vi "AlliGator Batch Dataset Export Window.vi"() -> ()   [LabVIEW 2021, in "AlliGator Files.lvlib"]
doc: "GUI for batch .ptu datasets export to HDF5 files or folders of TIFF images."
uses:
  AlliGator Files.lvlib
  AlliGator Batch File Conversion Item.ctl
  AlliGator Data Load & Process Options.ctl
  AlliGator Data Information.ctl
  AlliGator Gates to Skip.ctl
  AlliGator Define Gates to.ctl
  AlliGator Gates to Keep.ctl
  AlliGator Gate Arithmetic.ctl
  AlliGator Source Image Settings.ctl
  AlliGator Low Count Pixels Rejection Options.ctl
  AlliGator High Count Pixels Rejection Options.ctl
  AlliGator Image Smoothing Options.ctl
  Arrays/Kernel Type.ctl
  Arrays/Smoothing Algorithm.ctl
  AlliGator Image Binning Options.ctl
  AlliGator Decay Preprocessing Options.ctl
  AlliGator Background Subtraction Parameters.ctl
  AlliGator Baseline Subtraction Method.ctl
  AlliGator Decay Preprocessing Parameters.ctl
  Graphs/XY Graph/XY Graph Plot Shift Parameters.ctl
  Graphs/XY Graph/XY Graph Plot Shift Method.ctl
  <vilib>/Averna/BalloonTip/BalloonTip.llb/BalloonIcon.ctl
  <vilib>/Utility/miscctls.llb/LVPoint32TypeDef.ctl
  <vilib>/Averna/BalloonTip/BalloonTip.llb/OriginPosition.ctl
  AlliGator Variables List.ctl
  AlliGator TIFF Series Options.ctl
  AlliGator Saved TIFF Image Type.ctl
  <vilib>/Averna/BalloonTip/BalloonTip.llb/SetCoords.vi
  835454da-008c-4cc5-9e1e-46d3d2ae4ada.vi
  <vilib>/Averna/BalloonTip/BalloonTip.llb/SetTitle.vi
  <vilib>/Averna/BalloonTip/BalloonTip.llb/SetText.vi
  <vilib>/Averna/BalloonTip/BalloonTip.llb/GetClickEvent.vi
  <vilib>/Averna/BalloonTip/BalloonTip.llb/SetClosable.vi
  <vilib>/Averna/BalloonTip/BalloonTip.llb/SetRoundCorner.vi
  <vilib>/Averna/BalloonTip/BalloonTip.llb/SetBalloonColor.vi
  <vilib>/Averna/BalloonTip/BalloonTip.llb/SetBalloonIcon.vi
  <vilib>/Averna/BalloonTip/BalloonTip.llb/SetCtlRefnum.vi
  <vilib>/Averna/BalloonTip/BalloonTip.llb/SetCtlOriginPosition.vi
  <vilib>/Averna/BalloonTip/BalloonTip.llb/Constructor.vi
  <vilib>/Averna/BalloonTip/BalloonTip.llb/GetDVR.vi
  Variant/Variant to Data/Variant to Boolean.vi
  <userlib>/_OpenG.lib/array/array.llb/Filter 1D Array with Scalar (Boolean)__ogtk.vi
  <userlib>/_OpenG.lib/array/array.llb/Delete Elements from 1D Array (Variant)__ogtk.vi
  <vilib>/ErrorRing/Error Ring.xnode
  GUI/GUI.lvlib
  <userlib>/_OpenG.lib/array/array.llb/openg_array.lvlib
  AlliGator Scripts.lvlib
  AlliGator Decay Analysis.lvlib
  AlliGator Settings.lvlib
  Arrays/Arrays.lvlib
  AlliGator Source Image.lvlib
  AlliGator Decay Preprocessing.lvlib
  Graphs/XY Graph/XY Graph Add-Ons.lvlib
  Notebook/Notebook.lvlib
  Rich Text Box/Rich Text Box.lvlib
  Strings/Strings.lvlib
  AlliGator Globals, Variables & Constants.lvlib
  Variant/Variant to Data/Variant to Data.lvlib
  <vilib>/Averna/BalloonTip/BalloonTip.llb/BalloonTip.lvclass
  Error/Error.lvlib
  Sound/Sound.lvlib
panel:
  out "Conversion Jobs":cluster{"File Path":path, "Exported":bool}[](array[cluster])
  out "Message":string
  out "Animated Busy Icon":bool=TRUE
  in  "Abort":bool
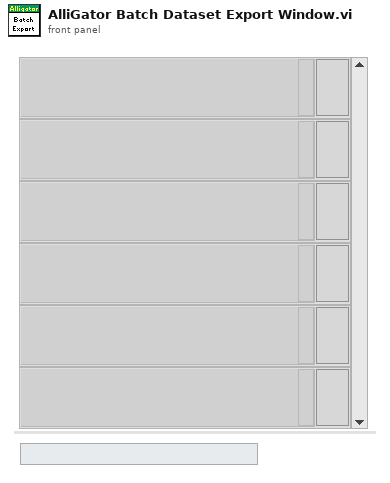
[diagram p1: front panel]
types:
  T1 = enum32{"Invalid", "Standard", "Closed", "Hidden", "Minimized", "Maximized"}
  T2 = typedef "AlliGator Globals, Variables & Constants.lvlib/AlliGator Variables List.ctl" = enum16{"---- GUI ----", "Initialization Status", "State Indicators Refnum", "Original AlliGator Menu Items", "Current Action Loop State", "Script in progress", "Playback", "Loop Playback", "Search ROI Used", "Search ROI", "Decay Graph Max Legend Size", "Intensity Graph Max Legend Size", "Decay Statistics Graph Max Legend Size", "Phasor Graph Max Legend Size", "Phasor Ratio Graph Max Legend Size", "Lifetime Graph Max Legend Size", "---- Files ----", "Export Dataset Frames as Individual Files", "Show Batch Export Help Balloons", "Frames in Dataset", "ptu File Frame Start Indices", "Current Frame in Dataset", "Current Frame Timestamp", "------ Python Plugins ------", "Python Plugins Information", "Python Session", "Valid Python Session?", "---- Source Image ----", "Dataset Loaded", "Dataset Metadata", "Dataset Channel", "Dataset Data Description", "Background Dataset Metadata", "Background Dataset Channel", "Background Dataset Data Description", "Background File Subtraction", "Background File Path", "Background File Pile-up Correction", "Background File Pixel Well Capacity", "Background File Scaling Factor", "Source Image ROIs", "Current Source Image ROI", "Source Image ROI Event Refnum", "X_Source Image Display Range", "X_Source Image Palette Information", "Source Image Palette List", "Source Image Scale", "Current Dataset Load Settings", "Source Image:ROI Overlay Color", "---- Image Profile Window ----", "Image Profile:Overlay ROI in Source Image", "Image Profile Window Event Refnum", "Image Profile:IntensityType", "Image Profile:Intensity Average Type", "Image Profile:Intensity-weighted SDV", "Image Profile:Box Profile Type", "Image Profile Window Open", "Image Profile:Plotted Fit Parameter", "X_Type of Displayed Image", "X_Time Gate Slider", "Dataset Path", "Source Image Overlay to Erase", "Is Displayed Image Accumulated", "White Light Image Modified", "Mask Image Modified", "Macrotime Gate Separation", "------ Phasor Graph -------", "Phasor Graph:Show Line", "---- Phasor Plot ---", "Phasor Plot Parameters Changed", "FLI Dataset Modified since last Phasor Plot Calculation", "Phasor Harmonics Data", "Selected Phasor Harmonics", "Phasor Harmonic Manager Event Refnum", "Phasor Plot ROIs", "Current Phasor Plot ROI", "Phasor Plot ROI Event Refnum", "Phasor Plot Image Reference Points", "Phasor Plot Computed", "Phasor Plot Palette Information", "Phasor Plot Palette List", "Phasor Ratio Palette Information", "Phasor Ratio Palette List", "Phasor Image Scale", "Phasor Plot Image Overlay to Erase", "Phasor Plot Image Elements to Update", "Current Phasor Plot Calculation Parameters", "Current Phasor Calibration Options", "Reset Cumulated Phasor Plot", "Phasor Ratio Reference 1", "Phasor Ratio Lifetime Reference 1", "Phasor Ratio Reference 1 Frequency", "Phasor Ratio Reference 2", "Phasor Ratio Lifetime Reference 2", "Phasor Ratio Reference 2 Frequency", "---- Decay Analysis ----", "Number of Selected Decays to Fit", "LS Fit Results", "LAR Fit Results", "BS Fit Results", "Last Decay Max - Min", "Best Fit Parameters", "Best Fit Parameter Names", "Actual Size X", "Actual Size Y", "Binning X", "Binning Y", "Actual # Gates", "Dataset Number", "Gates to...", "Gates Skipped", "Gates to keep", "Gate Step", "Gate Separation", "Reversed Gates", "Pile-up Correction", "Pixel Well Capacity", "Background Subtracted", "Background Subtraction Method", "Background Definition Range", "Background File (deprecated)", "Number of Dataset Accumulated", "Array of Accumulated Dataset Paths", "Do Averaged Datasets", "Destination File Path", "Process Plot Target", "Use 1/D as Phasor Frequency", "---- Decay Fit Parameter Map -----", "Decay Fit Parameter Map Palette Information", "Decay Fit Parameter Map Palette List", "Local Decay Graph Window Event Refnum", "------- Local Decay Window ---------", "Use normalized IRF for convolution", "----- Miscellaneous ----", "Skippable Dialog Windows Status"}
  T3 = typedef "BalloonTip.lvlib/BalloonTip.lvclass/OriginPosition.ctl" = enum16{"TopLeft", "TopRight", "BottomLeft", "BottomRight"}
  T4 = typedef "LVPoint32TypeDef.ctl" = cluster{"Horizontal":i32, "Vertical":i32}
  T5 = typedef "BalloonTip.lvlib/BalloonTip.lvclass/BalloonIcon.ctl" = enum16{"None", "Information", "Warning", "Error"}
  T6 = typedef "AlliGator Scripts.lvlib/AlliGator Data Load & Process Options.ctl" = cluster{"Data Information":T7, "Source Image Settings":T12, "Decay Preprocessing Options & Parameters":T19, "Clear Phasor Graph":bool}
  T7 = typedef "AlliGator Scripts.lvlib/AlliGator Data Information.ctl" = cluster{"Gates to Skip":T8, "# Gates":u32, "Gate Step":u32, "Gate Duration":dbl[unit], "Gate Separation":dbl[unit], "Pile-up Correction":bool, "Pixel Well Capacity":u32, "Define Gates to":T9, "Gates to Keep":T10, "Laser Period":dbl[unit], "SYNC Period":dbl[unit], "Channel Name":u16, "Channel Arithmetic":T11, "Background File Subtraction":bool, "Background Scaling Factor":dbl, "Background File":path, "Background Pile-up Correction":bool, "Background Pixel Well Capacity":u32, "Dataset Scaling Factor":dbl}
  T8 = typedef "AlliGator Decay Analysis.lvlib/AlliGator Gates to Skip.ctl" = cluster{"Start":u32, "End":u32}
  T9 = typedef "AlliGator Settings.lvlib/AlliGator Define Gates to.ctl" = enum32{"Skip", "Keep"}
  T10 = typedef "AlliGator Settings.lvlib/AlliGator Gates to Keep.ctl" = cluster{"First":u32, "Last":u32}
  T11 = typedef "AlliGator Settings.lvlib/AlliGator Gate Arithmetic.ctl" = enum16{"None", "INT-G2", "G2/INT*<INT>", "(1 - G2/INT)*<INT>"}
  T12 = typedef "AlliGator Scripts.lvlib/AlliGator Source Image Settings.ctl" = cluster{"Low Count Pixels Rejection Options":T13, "High Count Pixels Rejection Options":T14, "Peak Threshold":dbl, "Intensity Threshold":dbl, "Image Smoothing Options":T15, "Image Binning Options":T18}
  T13 = typedef "AlliGator Settings.lvlib/AlliGator Low Count Pixels Rejection Options.ctl" = cluster{"Background Low Threshold Factor":dbl, "Fixed Low Background Threshold":dbl, "Reject Low Count Pixels":bool, "Low Percentile":dbl}
  T14 = typedef "AlliGator Settings.lvlib/AlliGator High Count Pixels Rejection Options.ctl" = cluster{"Background High Threshold Factor":dbl, "Fixed High Background Threshold":dbl, "Reject High Count Pixels":bool, "High Percentile":dbl}
  T15 = typedef "AlliGator Settings.lvlib/AlliGator Image Smoothing Options.ctl" = cluster{"Use Image Smoothing":bool, "Kernel Type":T16, "Bin":i32, "Algorithm":T17}
  T16 = typedef "Arrays.lvlib/Kernel Type.ctl" = enum16{"Uniform", "Bilinear", "Gaussian"}
  T17 = typedef "Arrays.lvlib/Smoothing Algorithm.ctl" = enum16{"Rapid", "Thorough"}
  T18 = typedef "AlliGator Source Image.lvlib/AlliGator Image Binning Options.ctl" = cluster{"Use Image Binning":bool, "X Bin":i32, "Y Bin":i32}
  T19 = typedef "AlliGator Decay Analysis.lvlib/AlliGator Decay Preprocessing.lvlib/AlliGator Decay Preprocessing Options.ctl" = cluster{"Background Subtraction Parameters":T20, "Decay Preprocessing Parameters":T22, "Preprocessing Steps Order":string[]}
  T20 = typedef "AlliGator Decay Analysis.lvlib/AlliGator Decay Preprocessing.lvlib/AlliGator Background Subtraction Parameters.ctl" = cluster{"Background Definition Range":cluster{"Min Gate":dbl[unit], "Max Gate":dbl[unit]}, "Baseline Subtraction Method":T21, "Background Subtraction?":bool, "Background File":path, "Background Constant":dbl, "Background Scaling Factor":dbl, "Background Pile-up Correction":bool, "Background Pixel Well Capacity":u32}
  T21 = typedef "AlliGator Decay Analysis.lvlib/AlliGator Decay Preprocessing.lvlib/AlliGator Baseline Subtraction Method.ctl" = enum16{"Mean", "Min", "Square Gated Single-Exponential", "File", "Constant"}
  T22 = typedef "AlliGator Decay Analysis.lvlib/AlliGator Decay Preprocessing.lvlib/AlliGator Decay Preprocessing Parameters.ctl" = cluster{"Background Subtraction":bool, "Straighten Decay":bool, "Reverse Gates":bool, "1-Normalized Decay":bool, "Smoothen Decay":bool, "Smoothing Parameter":dbl, "Shift Decay":bool, "Decay Shift Parameters":T23, "Extrapolate Decay":bool, "Additional Points":u32, "Head Fraction":dbl, "Pixel-Normalize Decay":bool, "Use Periodicity":bool, "Use Cursors":bool, "Tail Fraction":dbl, "Use Decay Pre-Processing":bool, "Fold Decay":bool, "# Folds":u32, "[0-1]-Normalized Decay":bool}
  T23 = typedef "XY Graph Add-Ons.lvlib/XY Graph Plot Shift Parameters.ctl" = cluster{"Type":T24, "Shift":dbl[unit], "Threshold":dbl, "Rotate":bool}
  T24 = typedef "XY Graph Add-Ons.lvlib/XY Graph Plot Shift Method.ctl" = enum16{"Default", "CFD", "Threshold", "Cross-Correlation"}
  T25 = typedef "AlliGator Files.lvlib/AlliGator Batch File Conversion Item.ctl" = cluster{"File Path":path, "Saved":bool}
  T26 = typedef "LVRectTypeDef.ctl" = cluster{"Left":i16, "Top":i16, "Right":i16, "Bottom":i16}
  T27 = typedef "AlliGator Files.lvlib/AlliGator Saved TIFF Image Type.ctl" = enum16{"Single Gate", "Sum of All Gates", "Phasor"}
  T28 = typedef "AlliGator Files.lvlib/AlliGator TIFF Series Options.ctl" = cluster{"Gate Image File Name":string, "File Number Format":string, "Start Index":u32, "Save Metadata File":bool, "Compress Image":bool}
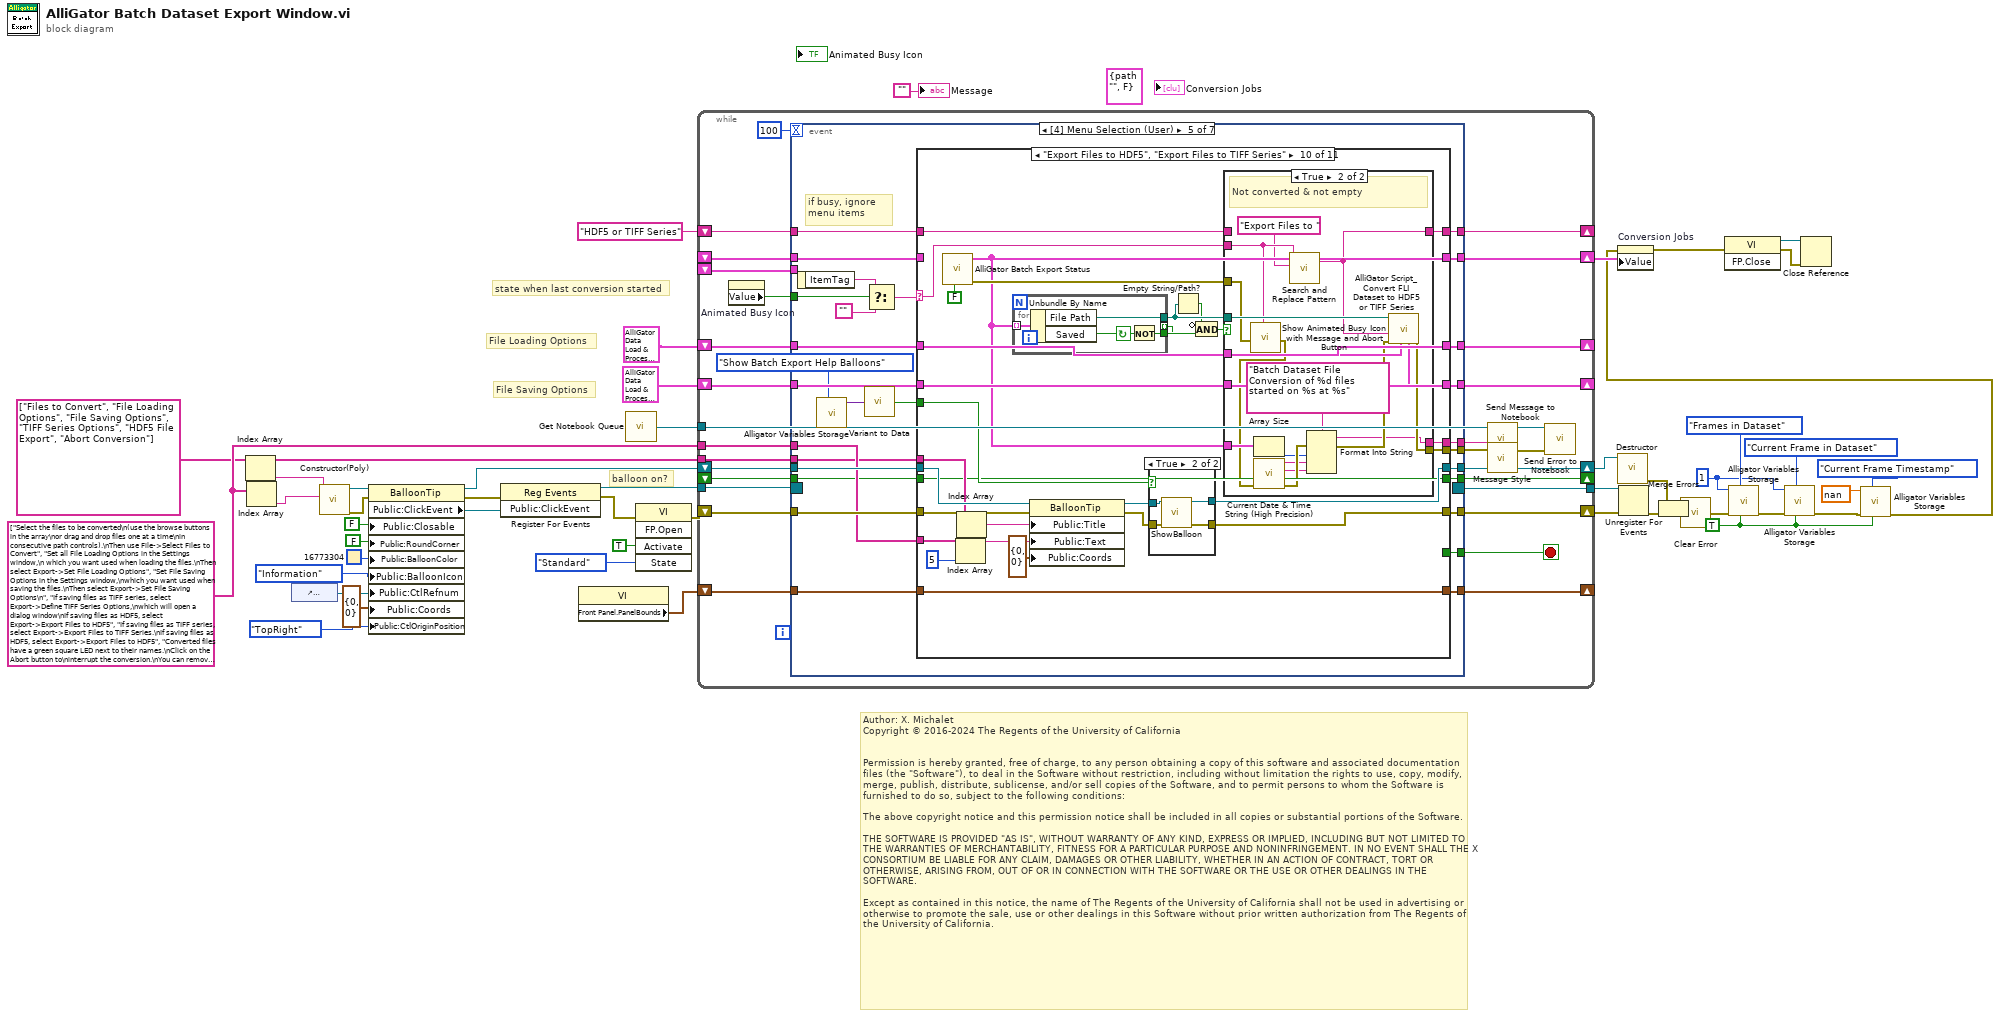
[diagram p0: block diagram]
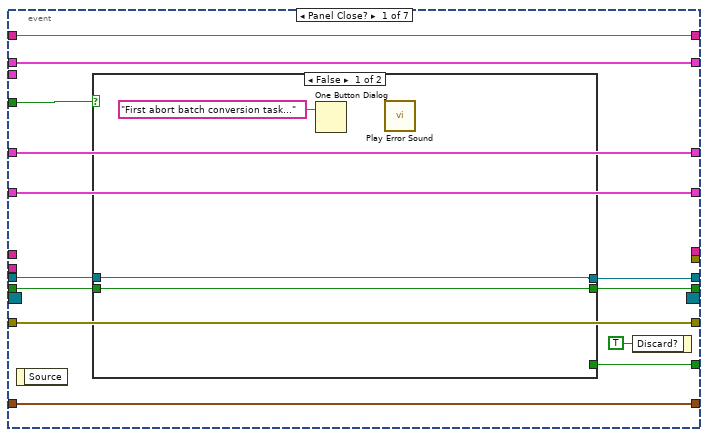
[diagram p2: hidden frame]
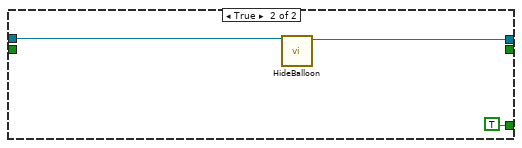
[diagram p3: hidden frame]
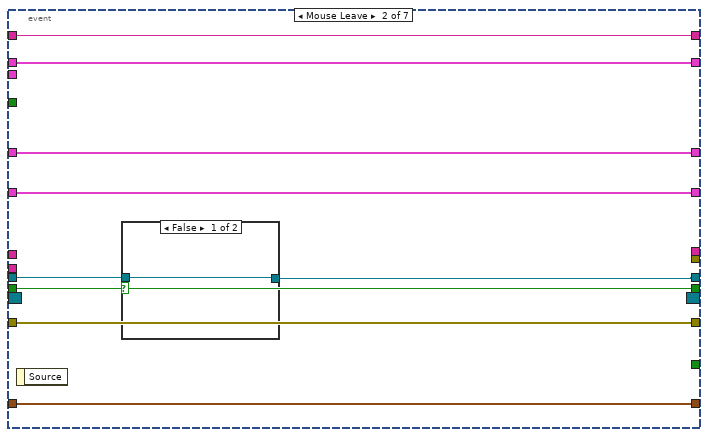
[diagram p4: hidden frame]
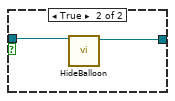
[diagram p5: hidden frame]
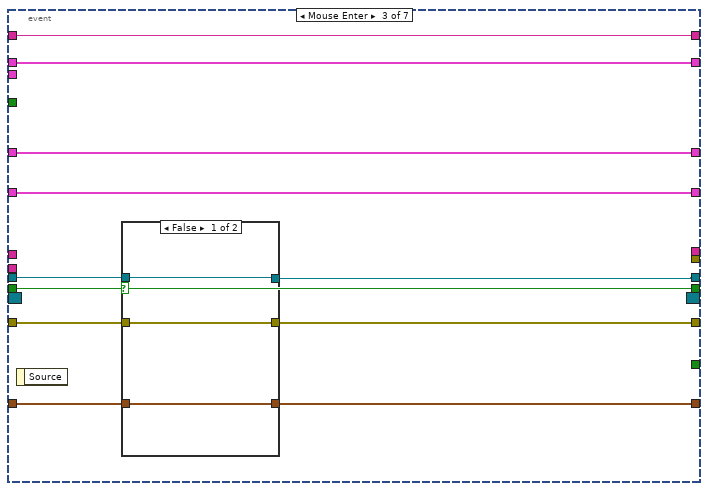
[diagram p6: hidden frame]
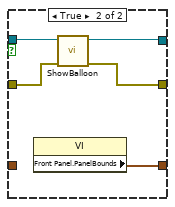
[diagram p7: hidden frame]
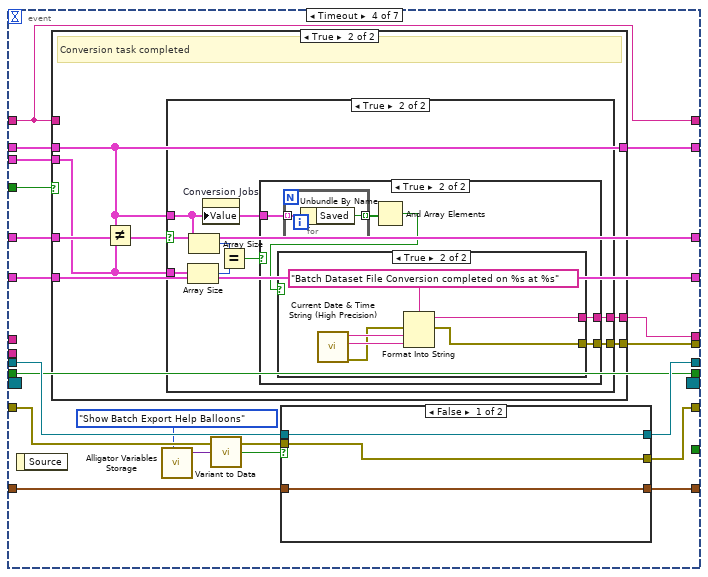
[diagram p8: hidden frame]
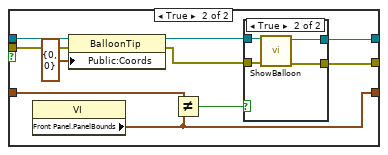
[diagram p9: hidden frame]
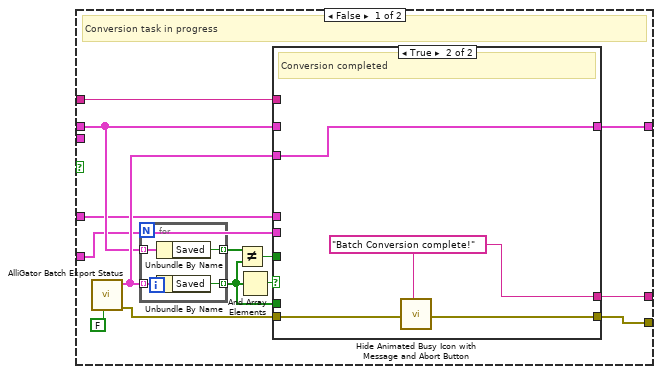
[diagram p11: hidden frame]
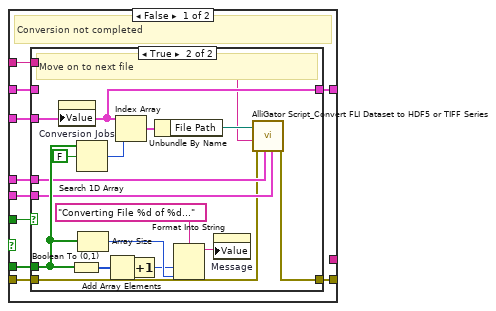
[diagram p12: hidden frame]
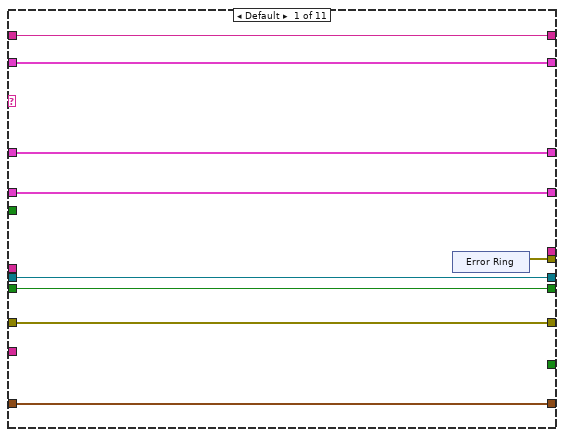
[diagram p17: hidden frame]
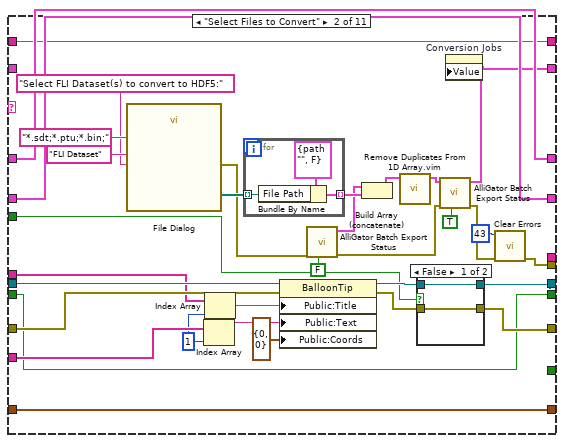
[diagram p18: hidden frame]
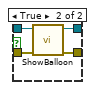
[diagram p19: hidden frame]
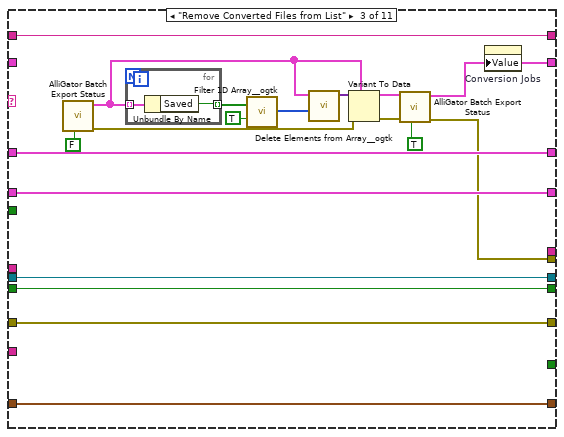
[diagram p20: hidden frame]
diagram:
  w14 = 1
  w11 = TRUE ("Get(F)/Set")
  w29 = string[] ["Files to Convert", "File Loading Options", "File Saving Options", "TIFF Series Options", "HDF5 File Export", "Abort Conversion"]
  w30 = string[] ["Select the files to be converted\n(use the browse buttons in the array\nor drag and drop files one at a time\nin consecutive path controls).\nThen use File->Select Files to Convert", "Set all File Loading Options in the Settings window,\n which you want used when loading the files.\nThen select Export->Set File Loading Options", "Set File Saving Options in the Settings window,\nwhich you want used when saving the files.\nThen select Export->Set File Saving Options\n", "If saving files as TIFF series, select Export->Define TIFF Series Options,\nwhich will open a dialog window\nIf saving files as HDF5, select Export->Export Files to HDF5", "If saving files as TIFF series, select Export->Export Files to TIFF Series.\nIf saving files as HDF5, select Export->Export Files to HDF5", "Converted files have a green square LED next to their names.\nClick on the Abort button to\ninterrupt the conversion.\nYou can remove the converted files\nfrom the list using File->Remove Converted Files from List."] ("Text")
  (unwired) T25 {"File Path"=path "", "Saved"=FALSE} ("File Array")
  # "Author: X. Michalet\nCopyright © 2016-2024 The Regents of the University of California\n \n\nPermission is hereby granted, free of charge, to any person obtaining a copy of this software and associated documentation files (the \"Software\"), to deal in the Software without restriction, including without limitation the rights to use, copy, modify, merge, publish, distribute, sublicense, and/or sell copies of the Software, and to permit persons to whom the Software is furnished to do so, subject to the following conditions:\n\nThe above copyright notice and this permission notice shall be included in all copies or substantial portions of the Software.\n\nTHE SOFTWARE IS PROVIDED \"AS IS\", WITHOUT WARRANTY OF ANY KIND, EXPRESS OR IMPLIED, INCLUDING BUT NOT LIMITED TO THE WARRANTIES OF MERCHANTABILITY, FITNESS FOR A PARTICULAR PURPOSE AND NONINFRINGEMENT. IN NO EVENT SHALL THE X CONSORTIUM BE LIABLE FOR ANY CLAIM, DAMAGES OR OTHER LIABILITY, WHETHER IN AN ACTION OF CONTRACT, TORT OR OTHERWISE, ARISING FROM, OUT OF OR IN CONNECTION WITH THE SOFTWARE OR THE USE OR OTHER DEALINGS IN THE SOFTWARE.\n\nExcept as contained in this notice, the name of The Regents of the University of California shall not be used in advertising or otherwise to promote the sale, use or other dealings in this Software without prior written authorization from The Regents of the University of California."
  # "balloon on?"
  # "File Saving Options"
  # "File Loading Options"
  # "state when last conversion started"
  n1 = Index Array(array=w29) -> (element=w25:string)  [unwired: 1 in]
  n2 = Index Array(array=w30) -> (element=w24:string)  [unwired: 1 in]
  n3 = control-ref of="Conversion Jobs"() -> (w28:refnum<vi>)
  n4 = call-poly <vilib>:"Constructor(Poly).vi"("Text"=w24, "Title (\"\")"=w25) -> ("error out"=w39:errorcluster, "BalloonTip out"=w40:refnum<class "BalloonTip.lvclass">)  [unwired: 8 in]
  n5 = property class="BalloonTip"(reference=w40, error in=w39, "Public:Closable"=FALSE ("Closable"), "Public:RoundCorner"=FALSE ("RoundCorner"), "Public:BalloonColor"=u32 16773304 ("BalloonColor"), "Public:BalloonIcon"=BalloonIcon."Information" ("BalloonIcon"), "Public:CtlRefnum"=w28, "Public:Coords"=T4 {"Horizontal"=0, "Vertical"=0} ("Coords"), "Public:CtlOriginPosition"=OriginPosition."TopRight" ("CtlOriginPosition")) -> (reference out=w38:refnum<class "BalloonTip.lvclass">, error out=w41:errorcluster, "Public:ClickEvent"=w2:refnum<user-event>)
  n6 = register-events(error in=w41, w2) -> (reference out=w37:refnum<event-registration>, error out=w5:errorcluster)  [unwired: 1 in]
  n7 = property class="VI"() -> ("Front Panel.PanelBounds"=w23:T26)  [unwired: 2 in, 2 out]
  n8 = call "Get Notebook Queue.vi"() -> ("Notebook Queue"=w1:refnum<queue>)  [unwired: 9 in]
  n9 = invoke class="VI" method="FP.Open"(error in=w5, "Activate"=TRUE ("Activate?"), "State"=T1."Standard") -> (error out=w6:errorcluster)  [unwired: 2 in, 4 out]
  n10 = while {
    shift-right: [w75] -> w46
    shift-left: _ -> [w73]
    shift-left: _ -> [w74]
    shift-right: [w72] -> _
    shift-left: T6 {"Data Information"={"Gates to Skip"={"Start"=0, "End"=0}, "# Gates"=1, "Gate Step"=1, "Gate Duration"=3e-10, "Gate Separation"=4e-11, "Pile-up Correction"=FALSE, "Pixel Well Capacity"=1, "Define Gates to"=enum."Skip", "Gates to Keep"={"First"=0, "Last"=0}, "Laser Period"=0.0, "SYNC Period"=0.0, "Channel Name"=0, "Channel Arithmetic"=enum."None", "Background File Subtraction"=FALSE, "Background Scaling Factor"=1.0, "Background File"=path "", "Background Pile-up Correction"=FALSE, "Background Pixel Well Capacity"=1, "Dataset Scaling Factor"=1.0}, "Source Image Settings"={"Low Count Pixels Rejection Options"={"Background Low Threshold Factor"=0.0, "Fixed Low Background Threshold"=20000.0, "Reject Low Count Pixels"=FALSE, "Low Percentile"=0.0}, "High Count Pixels Rejection Options"={"Background High Threshold Factor"=0.0, "Fixed High Background Threshold"=1.0, "Reject High Count Pixels"=FALSE, "High Percentile"=100.0}, "Peak Threshold"=500.0, "Intensity Threshold"=500.0, "Image Smoothing Options"={"Use Image Smoothing"=FALSE, "Kernel Type"=enum."Bilinear", "Bin"=1, "Algorithm"=enum."Rapid"}, "Image Binning Options"={"Use Image Binning"=FALSE, "X Bin"=1, "Y Bin"=1}}, "Decay Preprocessing Options & Parameters"={"Background Subtraction Parameters"={"Background Definition Range"={"Min Gate"=0.0, "Max Gate"=0.0}, "Baseline Subtraction Method"=enum."Mean", "Background Subtraction?"=FALSE, "Background File"=path "", "Background Constant"=0.0, "Background Scaling Factor"=1.0, "Background Pile-up Correction"=FALSE, "Background Pixel Well Capacity"=1}, "Decay Preprocessing Parameters"={"Background Subtraction"=FALSE, "Straighten Decay"=FALSE, "Reverse Gates"=FALSE, "1-Normalized Decay"=FALSE, "Smoothen Decay"=FALSE, "Smoothing Parameter"=0.0, "Shift Decay"=FALSE, "Decay Shift Parameters"={"Type"=enum."Default", "Shift"=0.0, "Threshold"=0.0, "Rotate"=FALSE}, "Extrapolate Decay"=FALSE, "Additional Points"=0, "Head Fraction"=0.0, "Pixel-Normalize Decay"=FALSE, "Use Periodicity"=FALSE, "Use Cursors"=FALSE, "Tail Fraction"=0.0, "Use Decay Pre-Processing"=TRUE, "Fold Decay"=FALSE, "# Folds"=1, "[0-1]-Normalized Decay"=FALSE}, "Preprocessing Steps Order"=[]}, "Clear Phasor Graph"=FALSE} ("Dataset Loading & Pre-processing Options (out)") -> [w71]
    shift-right: [w70] -> _
    shift-left: T6 {"Data Information"={"Gates to Skip"={"Start"=0, "End"=0}, "# Gates"=1, "Gate Step"=1, "Gate Duration"=3e-10, "Gate Separation"=4e-11, "Pile-up Correction"=FALSE, "Pixel Well Capacity"=1, "Define Gates to"=enum."Skip", "Gates to Keep"={"First"=0, "Last"=0}, "Laser Period"=0.0, "SYNC Period"=0.0, "Channel Name"=0, "Channel Arithmetic"=enum."None", "Background File Subtraction"=FALSE, "Background Scaling Factor"=1.0, "Background File"=path "", "Background Pile-up Correction"=FALSE, "Background Pixel Well Capacity"=1, "Dataset Scaling Factor"=1.0}, "Source Image Settings"={"Low Count Pixels Rejection Options"={"Background Low Threshold Factor"=0.0, "Fixed Low Background Threshold"=20000.0, "Reject Low Count Pixels"=FALSE, "Low Percentile"=0.0}, "High Count Pixels Rejection Options"={"Background High Threshold Factor"=0.0, "Fixed High Background Threshold"=1.0, "Reject High Count Pixels"=FALSE, "High Percentile"=100.0}, "Peak Threshold"=500.0, "Intensity Threshold"=500.0, "Image Smoothing Options"={"Use Image Smoothing"=FALSE, "Kernel Type"=enum."Bilinear", "Bin"=1, "Algorithm"=enum."Rapid"}, "Image Binning Options"={"Use Image Binning"=FALSE, "X Bin"=1, "Y Bin"=1}}, "Decay Preprocessing Options & Parameters"={"Background Subtraction Parameters"={"Background Definition Range"={"Min Gate"=0.0, "Max Gate"=0.0}, "Baseline Subtraction Method"=enum."Mean", "Background Subtraction?"=FALSE, "Background File"=path "", "Background Constant"=0.0, "Background Scaling Factor"=1.0, "Background Pile-up Correction"=FALSE, "Background Pixel Well Capacity"=1}, "Decay Preprocessing Parameters"={"Background Subtraction"=FALSE, "Straighten Decay"=FALSE, "Reverse Gates"=FALSE, "1-Normalized Decay"=FALSE, "Smoothen Decay"=FALSE, "Smoothing Parameter"=0.0, "Shift Decay"=FALSE, "Decay Shift Parameters"={"Type"=enum."Default", "Shift"=0.0, "Threshold"=0.0, "Rotate"=FALSE}, "Extrapolate Decay"=FALSE, "Additional Points"=0, "Head Fraction"=0.0, "Pixel-Normalize Decay"=FALSE, "Use Periodicity"=FALSE, "Use Cursors"=FALSE, "Tail Fraction"=0.0, "Use Decay Pre-Processing"=TRUE, "Fold Decay"=FALSE, "# Folds"=1, "[0-1]-Normalized Decay"=FALSE}, "Preprocessing Steps Order"=[]}, "Clear Phasor Graph"=FALSE} ("Dataset Loading & Pre-processing Options (out)") -> [w69]
    tunnel: w1 -> [w52]
    shift-right: [w68] -> _
    shift-left: "HDF5 or TIFF Series" ("result string") -> [w67]
    tunnel: w37 -> [w62]
    shift-right: [w61] -> w33
    shift-left: w38 -> [w63]
    tunnel: [w60] -> w32
    shift-right: [w59] -> w31
    shift-left: w6 -> [w64]
    tunnel: w30 -> [w58]
    tunnel: w29 -> [w57]
    shift-right: [w55] -> _
    shift-left: w23 -> [w56]
    shift-right: [w54] -> _
    shift-left: _ -> [w53]
    stop <- w65 stop-if-true
    n11 = property on="Animated Busy Icon" class="Bool (strict)"() -> ("Value"=w66:bool)  [unwired: 2 in, 2 out]
    n12 = event shown="[4] Menu Selection (User)" {
      selector: w62 -> [_ _ _ _ _ _ _]
      dyn-events: [_ _ _ _ _ _ _] -> w60
      timeout: 100 -> [_ _ _ _ _ _ _]
      tunnel: w66 -> [w89 _ _ w145 w268 _ _]
      tunnel: [w87 _ _ _ w266 _ _] -> w65
      tunnel: [w86 w104 w118 w143 w265 w567 w596] -> w75
      tunnel: w74 -> [w86 w104 w118 w144 w264 w567 w596]
      tunnel: w73 -> [_ _ _ w142 _ _ _]
      tunnel: [w85 w103 w117 w141 w261 w576 w595] -> w72
      tunnel: w71 -> [w85 w103 w117 w141 w260 w576 w595]
      tunnel: [w84 w102 w116 w140 w259 w575 w594] -> w70
      tunnel: w69 -> [w84 w102 w116 w140 w258 w575 w594]
      tunnel: [_ _ _ w139 w257 _ w592] -> w49
      tunnel: [w83 w101 w115 w138 w256 w574 w593] -> w68
      tunnel: w67 -> [w83 w101 w115 w138 w255 w574 w593]
      tunnel: w64 -> [w82 w100 w112 w134 w252 w559 w582]
      tunnel: w63 -> [w80 w98 w114 w135 w254 w560 w585]
      tunnel: [w79 w97 w113 w137 w253 w560 w584] -> w61
      tunnel: [w82 w100 w111 w136 w251 w559 w583] -> w59
      tunnel: w58 -> [_ _ _ _ w250 _ _]
      tunnel: w57 -> [_ _ _ _ w249 _ _]
      tunnel: w56 -> [w81 w99 w109 w130 w244 w558 w586]
      tunnel: [w81 w99 w110 w129 w245 w558 w586] -> w55
      tunnel: [w77 w96 w108 w128 w243 w557 w578] -> w54
      tunnel: w53 -> [w78 w96 w108 w128 w242 w557 w578]
      tunnel: [_ _ _ w127 w241 _ w577] -> w50
      event Panel Close? {
        n13 = event-data() -> ()  [unwired: 1 in, 1 out]
        n14 = case shown="False" w89 {
          tunnel: [_ TRUE ("Discard?")] -> w87
          tunnel: w80 -> [w91 w94]
          tunnel: [w91 w93] -> w79
          tunnel: w78 -> [w90 _]
          tunnel: [w90 _] -> w77
          frame False {
            n15 = One Button Dialog(message="First abort batch conversion task...") -> ()  [unwired: 1 in, 1 out]
            n16 = call "Play Error Sound.vi"() -> ()  [unwired: 27 in, 1 out]
          }
          frame True {
            n17 = call <vilib>:"HideBalloon.vi"("BalloonTip in"=w94) -> ("BalloonTip out"=w93:refnum<class "BalloonTip.lvclass">)  [unwired: 9 in, 1 out]
          }
        }
        n18 = event-data("Discard?"=TRUE) -> ()  [unwired: 1 in, 1 out]
      }
      event Mouse Leave {
        n19 = event-data() -> ()  [unwired: 1 in, 1 out]
        n20 = case shown="False" w96 {
          tunnel: w98 -> [w105 w107]
          tunnel: [w105 w106] -> w97
          frame False {
          }
          frame True {
            n21 = call <vilib>:"HideBalloon.vi"("BalloonTip in"=w107) -> ("BalloonTip out"=w106:refnum<class "BalloonTip.lvclass">)  [unwired: 9 in, 1 out]
          }
        }
      }
      event Mouse Enter {
        n22 = event-data() -> ()  [unwired: 1 in, 1 out]
        n23 = case shown="False" w108 {
          tunnel: w114 -> [w121 w125]
          tunnel: [w121 w126] -> w113
          tunnel: w112 -> [w119 w124]
          tunnel: [w119 w123] -> w111
          tunnel: [w120 w122] -> w110
          tunnel: w109 -> [w120 _]
          frame False {
          }
          frame True {
            n24 = property class="VI"() -> ("Front Panel.PanelBounds"=w122:T26)  [unwired: 2 in, 2 out]
            n25 = call <vilib>:"ShowBalloon.vi"("error in (no error)"=w124, "BalloonTip in"=w125) -> ("error out"=w123:errorcluster, "BalloonTip out"=w126:refnum<class "BalloonTip.lvclass">)  [unwired: 8 in]
          }
        }
      }
      event Timeout {
        n26 = event-data() -> ()  [unwired: 1 in, 1 out]
        n27 = case shown="True" w145 {
          tunnel: w144 -> [w173 w219]
          tunnel: [w175 w219] -> w143
          tunnel: w142 -> [_ w217]
          tunnel: w141 -> [w169 _]
          tunnel: w140 -> [w168 _]
          tunnel: [w167 w218] -> w139
          tunnel: w138 -> [w166 _]
          tunnel: [w165 w216] -> w127
          frame False {
            # "Conversion task in progress"
            n28 = call "AlliGator Batch Export Status.vi"("Set/Get (F)"=FALSE) -> ("error out"=w176:errorcluster, "Conversion Jobs out"=w174:T25[])  [unwired: 9 in]
            n29 = for {
              tunnel: w174 -> [w182] mode=indexing
              tunnel: [w181] -> w171 mode=indexing
              tunnel: w173 -> [w180] mode=indexing
              tunnel: [w179] -> w172 mode=indexing
              n30 = Unbundle By Name(w180) -> ("Saved"=w179:bool)
              n31 = Unbundle By Name(w182) -> ("Saved"=w181:bool)
            }
            n32 = Not Equal?(x=w172, y=w171) -> (x != y?=w170:bool)
            n33 = And Array Elements(Boolean array=w171) -> (logical AND=w177:bool)
            n34 = case shown="True" w177 {
              tunnel: w171 -> [w192 _]
              tunnel: w176 -> [w185 w215]
              tunnel: [w189 w214] -> w175
              tunnel: w174 -> [w188 w214]
              tunnel: w173 -> [w190 _]
              tunnel: w170 -> [w191 _]
              tunnel: w169 -> [w187 _]
              tunnel: w168 -> [w186 _]
              tunnel: [w184 w213] -> w167
              tunnel: w166 -> [w183 _]
              tunnel: [_ w212] -> w165
              frame False {
                # "Conversion not completed"
                n35 = case shown="True" w191 {
                  tunnel: w192 -> [_ w205]
                  tunnel: w190 -> [w194 _]
                  tunnel: [w194 w200] -> w189
                  tunnel: w188 -> [_ w200]
                  tunnel: w187 -> [_ w199]
                  tunnel: w186 -> [_ w198]
                  tunnel: w185 -> [w193 w197]
                  tunnel: [w193 w196] -> w184
                  tunnel: w183 -> [_ w195]
                  frame False {
                    # "conversion not complete"
                  }
                  frame True {
                    # "Move on to next file"
                    n36 = property on="Conversion Jobs" class="Arr"("Value"=w200) -> ()  [unwired: 2 in, 2 out]
                    n37 = Boolean To (0,1)(Boolean=w205) -> (0, 1=w211:i16[])
                    n38 = Search 1D Array(1D array=w205, element=FALSE) -> (index of element=w203:i32)  [unwired: 1 in]
                    n39 = Array Size(array=w205) -> (size(s)=w209:i32)
                    n40 = Add Array Elements(numeric array=w211) -> (sum=w210:i16)
                    n41 = Index Array(array=w200, index=w203) -> (element=w202:T25)
                    n42 = Increment(x=w210) -> (x+1=w206:i16)
                    n43 = Unbundle By Name(w202) -> ("File Path"=w201:path)
                    n44 = Format Into String(format string="Converting File %d of %d...", w206, w209) -> (resulting string=w207:string)  [unwired: 2 in, 1 out]
                    n45 = property on="Message" class="Str"("Value"=w207) -> ()  [unwired: 2 in, 2 out]
                    n46 = call "AlliGator Script_Convert FLI Dataset to HDF5 or TIFF Series.vi"("Dataset Saving Options"=w198, "Dataset Loading Options"=w199, "Error In"=w197, "Destination File Type"=w195, "File Path"=w201) -> ("Error Out"=w196:errorcluster)  [unwired: 6 in]
                  }
                }
              }
              frame True {
                w212 = "Batch Conversion complete!" ("Message")
                # "Conversion completed"
                n47 = call "Hide Animated Busy Icon with Message and Abort Button.vi"("Message"=w212, "Error In"=w215) -> ("Error Out"=w213:errorcluster)  [unwired: 17 in]
              }
            }
          }
          frame True {
            # "Conversion task completed"
            n48 = Not Equal?(x=w219, y=w217) -> (x != y?=w220:bool)
            n49 = case shown="True" w220 {
              tunnel: w219 -> [_ w222]
              tunnel: [_ w227] -> w218
              tunnel: w217 -> [_ w226]
              tunnel: [_ w221] -> w216
              frame False {
              }
              frame True {
                n50 = Array Size(array=w226) -> (size(s)=w224:i32)
                n51 = Array Size(array=w222) -> (size(s)=w225:i32)
                n52 = property on="Conversion Jobs" class="Arr"("Value"=w222) -> ()  [unwired: 2 in, 2 out]
                n53 = Equal?(x=w225, y=w224) -> (x = y?=w223:bool)
                n54 = case shown="True" w223 {
                  tunnel: [_ w232] -> w227
                  tunnel: w222 -> [_ w231]
                  tunnel: [_ w228] -> w221
                  frame False {
                  }
                  frame True {
                    n55 = for {
                      tunnel: w231 -> [w240] mode=indexing
                      tunnel: [w239] -> w230 mode=indexing
                      n56 = Unbundle By Name(w240) -> ("Saved"=w239:bool)
                    }
                    n57 = And Array Elements(Boolean array=w230) -> (logical AND=w229:bool)
                    n58 = case shown="True" w229 {
                      tunnel: [_ w234] -> w232
                      tunnel: [_ w233] -> w228
                      frame False {
                      }
                      frame True {
                        n59 = call "Current Date & Time String (High Precision).vi"() -> ("Error Out"=w236:errorcluster, "time string"=w237:string, "date string"=w238:string)  [unwired: 8 in, 1 out]
                        n60 = Format Into String(format string="Batch Dataset File Conversion completed on %s at %s", error in=w236, w238, w237) -> (resulting string=w233:string, error out=w234:errorcluster)  [unwired: 1 in]
                      }
                    }
                  }
                }
              }
            }
          }
        }
        n61 = call "Alligator Variables Storage.vi"("AlliGator Variable"=AlliGator_Variables_List."Show Batch Export Help Balloons" ("Alligator Variable")) -> ("Data out"=w133:variant)  [unwired: 8 in, 2 out]
        n62 = call-poly "Variant to Data.vi"("Variant"=w133) -> ("Value"=w132:bool)  [unwired: 8 in]
        n63 = case shown="False" w132 {
          tunnel: [w148 w152] -> w137
          tunnel: [w147 w151] -> w136
          tunnel: w135 -> [w148 w158]
          tunnel: w134 -> [w147 w157]
          tunnel: w130 -> [w146 w155]
          tunnel: [w146 w149] -> w129
          frame False {
          }
          frame True {
            n64 = property class="VI"() -> ("Front Panel.PanelBounds"=w149:T26)  [unwired: 2 in, 2 out]
            n65 = property class="BalloonTip"(reference=w158, error in=w157, "Public:Coords"=T4 {"Horizontal"=0, "Vertical"=0} ("Coords")) -> (reference out=w154:refnum<class "BalloonTip.lvclass">, error out=w153:errorcluster)
            n66 = Not Equal?(x=w155, y=w149) -> (x != y?=w150:bool)
            n67 = case shown="True" w150 {
              tunnel: w154 -> [w160 w164]
              tunnel: w153 -> [w159 w163]
              tunnel: [w160 w162] -> w152
              tunnel: [w159 w161] -> w151
              frame False {
              }
              frame True {
                n68 = call <vilib>:"ShowBalloon.vi"("error in (no error)"=w163, "BalloonTip in"=w164) -> ("error out"=w161:errorcluster, "BalloonTip out"=w162:refnum<class "BalloonTip.lvclass">)  [unwired: 8 in]
              }
            }
          }
        }
      }
      event Menu Selection (User) {
        # "if busy, ignore menu items"
        n69 = event-data() -> ("ItemTag"=w263:string)  [unwired: 1 in]
        n70 = call "Alligator Variables Storage.vi"("AlliGator Variable"=AlliGator_Variables_List."Show Batch Export Help Balloons" ("Alligator Variable")) -> ("Data out"=w248:variant)  [unwired: 8 in, 2 out]
        n71 = call-poly "Variant to Data.vi"("Variant"=w248) -> ("Value"=w246:bool)  [unwired: 8 in]
        n72 = Select(t=w263, s=w268, f="") -> (s? t:f=w267:string)
        n73 = case shown="\"Export Files to HDF5\", \"Export Files to TIFF Series\"" w267 {
          selector: w267 -> [_ _ _ _ _ _ _ _ _ w505 _]
          tunnel: [_ _ _ _ _ _ _ _ _ _ TRUE] -> w266
          tunnel: [w277 w279 w322 w361 w384 w401 w431 w470 w485 w506 w554] -> w265
          tunnel: w264 -> [w277 _ _ w361 w384 w401 w431 w470 _ _ w554]
          tunnel: [w276 w307 w330 w362 w383 w400 w429 w469 w484 w509 w553] -> w261
          tunnel: w260 -> [w276 w307 w330 _ w383 w400 w429 w469 w484 w509 w553]
          tunnel: [w275 w308 w329 w360 w382 w399 w430 w468 w483 w508 w552] -> w259
          tunnel: w258 -> [w275 w308 w329 w360 w382 w399 _ w468 w483 w508 w552]
          tunnel: [w269 w296 w328 w359 w370 w385 w428 w439 w482 w507 w545] -> w257
          tunnel: [w274 w304 w327 w358 w381 w398 w427 w456 w481 w504 w551] -> w256
          tunnel: w255 -> [w274 w304 w327 w358 w381 w398 w427 w456 w481 w503 w551]
          tunnel: w254 -> [w273 w294 w326 w354 w374 w392 w423 w452 w480 w499 w548]
          tunnel: [w273 w285 w326 w347 w374 w391 w416 w445 w480 w491 w547] -> w253
          tunnel: w252 -> [w272 w293 w325 w353 w373 w390 w422 w451 w479 w498 w550]
          tunnel: [w272 w284 w325 w348 w373 w389 w417 w446 w479 w492 w550] -> w251
          tunnel: w250 -> [_ w292 _ w351 _ _ w420 w449 _ w496 _]
          tunnel: w249 -> [_ w288 _ w352 _ _ w421 w450 _ w497 _]
          tunnel: w246 -> [_ w283 _ w346 _ _ w414 w444 _ w490 _]
          tunnel: [w271 w281 w324 w344 w372 w388 w413 w442 w478 w489 w549] -> w245
          tunnel: w244 -> [w271 w281 w324 w344 w372 w387 w413 w442 w478 w489 w549]
          tunnel: [w270 w280 w323 w343 w371 w386 w412 w441 w477 w488 w546] -> w243
          tunnel: w242 -> [w270 w280 w323 w343 w371 _ w412 w441 w477 w488 w546]
          tunnel: [_ _ _ _ _ _ _ _ _ w487 _] -> w241
          frame Default {
            n74 = xnode "Error Ring"() -> ("error out"=w269:errorcluster)
          }
          frame "Select Files to Convert" {
            w289 = 1 ("index")
            n75 = call "File Dialog"("prompt"="Select FLI Dataset(s) to convert to HDF5:", "pattern (all files)"="*.sdt;*.ptu;*.bin;", "pattern label"="FLI Dataset") -> ("selected paths"=w309:path[], "error out"=w306:errorcluster)  [unwired: 9 in, 2 out]
            n76 = Index Array(array=w292, index=w289) -> (element=w291:string)
            n77 = Index Array(array=w288, index=w289) -> (element=w290:string)
            n78 = for {
              tunnel: w309 -> [w320] mode=indexing
              tunnel: [w321] -> w303 mode=indexing
              n79 = Bundle By Name(cluster=T25 {"File Path"=path "", "Saved"=FALSE} ("File Array"), "File Path"=w320) -> (w321:T25)
            }
            n80 = property class="BalloonTip"(reference=w294, error in=w293, "Public:Title"=w290, "Public:Text"=w291, "Public:Coords"=T4 {"Horizontal"=0, "Vertical"=0} ("Coords")) -> (reference out=w287:refnum<class "BalloonTip.lvclass">, error out=w286:errorcluster)
            n81 = call "AlliGator Batch Export Status.vi"("Set/Get (F)"=FALSE, "error in (no error)"=w306) -> ("error out"=w297:errorcluster, "Conversion Jobs out"=w301:T25[])  [unwired: 8 in]
            n82 = Build Array (concatenate)(w301, w303) -> (w302:T25[])
            n83 = call "Remove Duplicates From 1D Array.vim"("array"=w302) -> ("array with duplicates removed"=w299:T25[])  [unwired: 10 in]
            n84 = case shown="False" w283 {
              tunnel: w287 -> [w314 w318]
              tunnel: w286 -> [w313 w317]
              tunnel: [w314 w316] -> w285
              tunnel: [w313 w315] -> w284
              frame False {
              }
              frame True {
                n85 = call <vilib>:"ShowBalloon.vi"("error in (no error)"=w317, "BalloonTip in"=w318) -> ("error out"=w315:errorcluster, "BalloonTip out"=w316:refnum<class "BalloonTip.lvclass">)  [unwired: 8 in]
              }
            }
            n86 = call "AlliGator Batch Export Status.vi"("Set/Get (F)"=TRUE, "error in (no error)"=w297, "Conversion Jobs in"=w299) -> ("error out"=w305:errorcluster, "Conversion Jobs out"=w279:T25[])  [unwired: 7 in]
            n87 = property on="Conversion Jobs" class="Arr"("Value"=w279) -> ()  [unwired: 2 in, 2 out]
            n88 = call <vilib>:"Clear Errors.vi"("error in (no error)"=w305, "specific error code to clear (0: all)"=43) -> ("error out"=w296:errorcluster)  [unwired: 4 in, 1 out]
          }
          frame "Remove Converted Files from List" {
            n89 = call "AlliGator Batch Export Status.vi"("Set/Get (F)"=FALSE) -> ("error out"=w331:errorcluster, "Conversion Jobs out"=w334:T25[])  [unwired: 9 in]
            n90 = for {
              tunnel: w334 -> [w342] mode=indexing
              tunnel: [w341] -> w340 mode=indexing
              n91 = Unbundle By Name(w342) -> ("Saved"=w341:bool)
            }
            n92 = call-poly <userlib>:"Filter 1D Array__ogtk.vi"("items to filter"=TRUE ("Boolean"), "array"=w340) -> ("filtered item indices"=w338:i32[])  [unwired: 4 in, 1 out]
            n93 = call-poly <userlib>:"Delete Elements from Array__ogtk.vi"("indices"=w338, "array"=w334) -> ("array w/ subset deleted"=w336:variant[])  [unwired: 8 in, 1 out]
            n94 = Variant To Data(error in=w331, type=w334, Variant=w336) -> (data=w335:T25[], error out=w332:errorcluster)
            n95 = call "AlliGator Batch Export Status.vi"("Set/Get (F)"=TRUE, "error in (no error)"=w332, "Conversion Jobs in"=w335) -> ("error out"=w328:errorcluster, "Conversion Jobs out"=w322:T25[])  [unwired: 7 in]
            n96 = property on="Conversion Jobs" class="Arr"("Value"=w322) -> ()  [unwired: 2 in, 2 out]
          }
          frame "Set File Loading Options" {
            w355 = 2 ("index")
            n97 = Index Array(array=w351, index=w355) -> (element=w357:string)
            n98 = Index Array(array=w352, index=w355) -> (element=w356:string)
            n99 = property class="BalloonTip"(reference=w354, error in=w353, "Public:Title"=w356, "Public:Text"=w357, "Public:Coords"=T4 {"Horizontal"=0, "Vertical"=0} ("Coords")) -> (reference out=w350:refnum<class "BalloonTip.lvclass">, error out=w349:errorcluster)
            n100 = call "AlliGator Get-Set Loading & Pre-Processing Options.vi"("Get (F)/Set"=FALSE) -> ("Error Out"=w359:errorcluster, "Dataset Loading & Pre-processing Options (out)"=w362:T6)  [unwired: 9 in]
            n101 = case shown="False" w346 {
              tunnel: w350 -> [w365 w369]
              tunnel: w349 -> [w364 w368]
              tunnel: [w364 w367] -> w348
              tunnel: [w365 w366] -> w347
              frame False {
              }
              frame True {
                n102 = call <vilib>:"ShowBalloon.vi"("error in (no error)"=w368, "BalloonTip in"=w369) -> ("error out"=w367:errorcluster, "BalloonTip out"=w366:refnum<class "BalloonTip.lvclass">)  [unwired: 8 in]
              }
            }
          }
          frame "Export .ptu Frames as Individual Files" {
            w380 = AlliGator_Variables_List."Export Dataset Frames as Individual Files" ("Alligator Variable")
            n103 = call "Alligator Variables Storage.vi"("AlliGator Variable"=w380) -> ("Error Out"=w379:errorcluster, "Data out"=w378:variant)  [unwired: 8 in, 1 out]
            n104 = call-poly "Variant to Data.vi"("Variant"=w378) -> ("Value"=w377:bool)  [unwired: 8 in]
            n105 = Not(x=w377) -> (.not. x?=w376:bool)
            n106 = call "Alligator Variables Storage.vi"("Get(F)/Set"=TRUE, "AlliGator Variable"=w380, "Error In"=w379, "Data in"=w376) -> ("Error Out"=w370:errorcluster)  [unwired: 5 in, 2 out]
          }
          frame "Show Help Balloons" {
            w397 = AlliGator_Variables_List."Show Batch Export Help Balloons" ("Alligator Variable")
            n107 = call "Alligator Variables Storage.vi"("AlliGator Variable"=w397) -> ("Error Out"=w396:errorcluster, "Data out"=w395:variant)  [unwired: 8 in, 1 out]
            n108 = call-poly "Variant to Data.vi"("Variant"=w395) -> ("Value"=w393:bool)  [unwired: 8 in]
            n109 = Not(x=w393) -> (.not. x?=w386:bool)
            n110 = case shown="False" w393 {
              tunnel: w392 -> [w406 w411]
              tunnel: [w405 w410] -> w391
              tunnel: w390 -> [w404 w409]
              tunnel: [w403 w408] -> w389
              tunnel: [w402 w407] -> w388
              tunnel: w387 -> [_ w407]
              frame False {
                n111 = property class="VI"() -> ("Front Panel.PanelBounds"=w402:T26)  [unwired: 2 in, 2 out]
                n112 = call <vilib>:"ShowBalloon.vi"("error in (no error)"=w404, "BalloonTip in"=w406) -> ("error out"=w403:errorcluster, "BalloonTip out"=w405:refnum<class "BalloonTip.lvclass">)  [unwired: 8 in]
              }
              frame True {
                n113 = call <vilib>:"HideBalloon.vi"("error in (no error)"=w409, "BalloonTip in"=w411) -> ("error out"=w408:errorcluster, "BalloonTip out"=w410:refnum<class "BalloonTip.lvclass">)  [unwired: 8 in]
              }
            }
            n114 = call "Alligator Variables Storage.vi"("Get(F)/Set"=TRUE, "AlliGator Variable"=w397, "Error In"=w396, "Data in"=w386) -> ("Error Out"=w385:errorcluster)  [unwired: 5 in, 2 out]
          }
          frame "Set File Saving Options" {
            w424 = 3 ("index")
            n115 = Index Array(array=w420, index=w424) -> (element=w426:string)
            n116 = Index Array(array=w421, index=w424) -> (element=w425:string)
            n117 = property class="BalloonTip"(reference=w423, error in=w422, "Public:Title"=w425, "Public:Text"=w426, "Public:Coords"=T4 {"Horizontal"=0, "Vertical"=0} ("Coords")) -> (reference out=w419:refnum<class "BalloonTip.lvclass">, error out=w418:errorcluster)
            n118 = case shown="False" w414 {
              tunnel: w419 -> [w434 w438]
              tunnel: w418 -> [w433 w437]
              tunnel: [w433 w436] -> w417
              tunnel: [w434 w435] -> w416
              frame False {
              }
              frame True {
                n119 = call <vilib>:"ShowBalloon.vi"("error in (no error)"=w437, "BalloonTip in"=w438) -> ("error out"=w436:errorcluster, "BalloonTip out"=w435:refnum<class "BalloonTip.lvclass">)  [unwired: 8 in]
              }
            }
            n120 = call "AlliGator Get-Set Loading & Pre-Processing Options.vi"("Get (F)/Set"=FALSE) -> ("Error Out"=w428:errorcluster, "Dataset Loading & Pre-processing Options (out)"=w430:T6)  [unwired: 9 in]
          }
          frame "Define TIFF Series Options" {
            w453 = 4 ("index")
            n121 = Index Array(array=w449, index=w453) -> (element=w455:string)
            n122 = Index Array(array=w450, index=w453) -> (element=w454:string)
            n123 = call "AlliGator Gate Image File Name Format Dialog.vi"("Single Image"=FALSE, "Saved TIFF Image"=AlliGator_Saved_TIFF_Image_Type."Single Gate", "Image File Name in"="(Leave empty to use original file name)") -> ("error out"=w463:errorcluster, "Start Index out"=w461:u32, "File Number Format out"=w464:string, "Gate Image File Name out"=w465:string, "Compress Image out"=w460:bool, "Save Metadata File out"=w459:bool)  [unwired: 2 in, 1 out]
            n124 = Bundle(cluster=T28 {"Gate Image File Name"="", "File Number Format"="", "Start Index"=0, "Save Metadata File"=FALSE, "Compress Image"=FALSE} ("output cluster"), "Gate Image File Name"=w465, "File Number Format"=w464, "Start Index"=w461, "Save Metadata File"=w460, "Compress Image"=w459) -> (w458:T28)
            n125 = property class="BalloonTip"(reference=w452, error in=w451, "Public:Title"=w454, "Public:Text"=w455, "Public:Coords"=T4 {"Horizontal"=0, "Vertical"=0} ("Coords")) -> (reference out=w448:refnum<class "BalloonTip.lvclass">, error out=w447:errorcluster)
            n126 = call "AlliGator Get-Set TIFF Series Options.vi"("Set/Get (F)"=TRUE, "error in (no error)"=w463, "output cluster in"=w458) -> ("error out"=w439:errorcluster)  [unwired: 7 in, 1 out]
            n127 = case shown="False" w444 {
              tunnel: w448 -> [w472 w476]
              tunnel: w447 -> [w471 w475]
              tunnel: [w471 w474] -> w446
              tunnel: [w472 w473] -> w445
              frame False {
              }
              frame True {
                n128 = call <vilib>:"ShowBalloon.vi"("error in (no error)"=w475, "BalloonTip in"=w476) -> ("error out"=w474:errorcluster, "BalloonTip out"=w473:refnum<class "BalloonTip.lvclass">)  [unwired: 8 in]
              }
            }
          }
          frame "Empty Conversion List" {
            w485 = T25[] [] ("Conversion Jobs in")
            n129 = call "AlliGator Batch Export Status.vi"("Set/Get (F)"=TRUE, "Conversion Jobs in"=w485) -> ("error out"=w482:errorcluster)  [unwired: 8 in, 1 out]
            n130 = property on="Conversion Jobs" class="Arr"("Value"=w485) -> ()  [unwired: 2 in, 2 out]
          }
          frame "Export Files to HDF5", "Export Files to TIFF Series" {
            w500 = 5 ("index")
            n131 = call "AlliGator Batch Export Status.vi"("Set/Get (F)"=FALSE) -> ("error out"=w514:errorcluster, "Conversion Jobs out"=w506:T25[])  [unwired: 9 in]
            n132 = Index Array(array=w496, index=w500) -> (element=w502:string)
            n133 = Index Array(array=w497, index=w500) -> (element=w501:string)
            n134 = for {
              tunnel: w506 -> [w544] mode=indexing
              tunnel: [w541] -> w512 if=w542
              tunnel: [w542] -> _ mode=indexing
              tunnel: [w542] -> w513
              stop <- w543 continue-if-true
              n135 = Unbundle By Name(w544) -> ("File Path"=w541:path, "Saved"=w543:bool)
              n136 = Not(x=w543) -> (.not. x?=w542:bool)
            }
            n137 = property class="BalloonTip"(reference=w499, error in=w498, "Public:Title"=w501, "Public:Text"=w502, "Public:Coords"=T4 {"Horizontal"=0, "Vertical"=0} ("Coords")) -> (reference out=w494:refnum<class "BalloonTip.lvclass">, error out=w493:errorcluster)
            n138 = case shown="True" w490 {
              tunnel: w494 -> [w517 w521]
              tunnel: w493 -> [w516 w520]
              tunnel: [w516 w519] -> w492
              tunnel: [w517 w518] -> w491
              frame False {
              }
              frame True {
                n139 = call <vilib>:"ShowBalloon.vi"("error in (no error)"=w520, "BalloonTip in"=w521) -> ("error out"=w519:errorcluster, "BalloonTip out"=w518:refnum<class "BalloonTip.lvclass">)  [unwired: 8 in]
              }
            }
            n140 = Empty String/Path?(string/path=w512) -> (empty?=w510:bool)
            n141 = Compound Arithmetic op=AND(invert w510, w513) -> (w511:bool)
            n142 = case shown="True" w511 {
              tunnel: w512 -> [_ w540]
              tunnel: w514 -> [w523 w528]
              tunnel: w509 -> [_ w539]
              tunnel: w508 -> [_ w538]
              tunnel: [w523 w525] -> w507
              tunnel: w506 -> [_ w532]
              tunnel: w505 -> [_ w531]
              tunnel: [w522 w529] -> w504
              tunnel: w503 -> [w522 _]
              tunnel: [_ w524] -> w487
              frame False {
                # "all files converted or no files"
              }
              frame True {
                # "Not converted & not empty"
                n143 = call "Show Animated Busy Icon with Message and Abort Button.vi"("Message"=w531, "Error In"=w528) -> ("Error Out"=w527:errorcluster)  [unwired: 17 in]
                n144 = Array Size(array=w532) -> (size(s)=w533:i32)
                n145 = call "Current Date & Time String (High Precision).vi"("Error In"=w527) -> ("Error Out"=w537:errorcluster, "time string"=w536:string, "date string"=w534:string)  [unwired: 7 in, 1 out]
                n146 = call <vilib>:"Search and Replace Pattern.vi"("string"=w531, "regular expression (\"\")"="Export Files to " ("regular expression (\"\")")) -> ("result string"=w529:string)  [unwired: 3 in, 1 out]
                n147 = Format Into String(format string="Batch Dataset File Conversion of %d files started on %s at %s", error in=w537, w533, w534, w536) -> (resulting string=w524:string, error out=w526:errorcluster)  [unwired: 1 in]
                n148 = call "AlliGator Script_Convert FLI Dataset to HDF5 or TIFF Series.vi"("Dataset Saving Options"=w538, "Dataset Loading Options"=w539, "Error In"=w526, "Destination File Type"=w529, "File Path"=w540) -> ("Error Out"=w525:errorcluster)  [unwired: 6 in]
              }
            }
          }
          frame "Close" {
            n149 = call <vilib>:"HideBalloon.vi"("BalloonTip in"=w548) -> ("BalloonTip out"=w547:refnum<class "BalloonTip.lvclass">)  [unwired: 9 in, 1 out]
            n150 = xnode "Error Ring"() -> ("error out"=w545:errorcluster)
          }
        }
      }
      event Menu Activation? {
        n151 = event-data() -> ("MenuRef"=w573:refnum<k9>)  [unwired: 1 in]
        n152 = call "Alligator Variables Storage.vi"("AlliGator Variable"=AlliGator_Variables_List."Show Batch Export Help Balloons" ("Alligator Variable")) -> ("Error Out"=w563:errorcluster, "Data out"=w564:variant)  [unwired: 8 in, 1 out]
        n153 = call "Alligator Variables Storage.vi"("AlliGator Variable"=AlliGator_Variables_List."Export Dataset Frames as Individual Files" ("Alligator Variable")) -> ("Error Out"=w568:errorcluster, "Data out"=w570:variant)  [unwired: 8 in, 1 out]
        n154 = call-poly "Variant to Data.vi"("Variant"=w564) -> ("Value"=w562:bool)  [unwired: 8 in]
        n155 = call-poly "Variant to Data.vi"("Variant"=w570) -> ("Value"=w569:bool)  [unwired: 8 in]
        n156 = Set Menu Item Info(6:w569, 7:"Export .ptu Frames as Individual Files" ("item tag"), 8:w568, 11:w573) -> (3:w566:refnum<k9>)  [unwired: 3 in, 1 out]
        n157 = Set Menu Item Info(6:w562, 7:"Show Help Balloons" ("item tag"), 8:w563, 11:w566) -> ()  [unwired: 3 in, 2 out]
        n158 = event-data() -> ()  [unwired: 2 in, 1 out]
      }
      event "Abort": Value Change {
        n159 = event-data() -> ()  [unwired: 1 in, 1 out]
        n160 = call <vilib>:"HideBalloon.vi"("error in (no error)"=w582, "BalloonTip in"=w585) -> ("error out"=w583:errorcluster, "BalloonTip out"=w584:refnum<class "BalloonTip.lvclass">)  [unwired: 8 in]
        n161 = call "Alligator Variables Storage.vi"("Get(F)/Set"=TRUE, "AlliGator Variable"=AlliGator_Variables_List."Show Batch Export Help Balloons" ("Alligator Variable"), "Data in"=FALSE ("Get(F)/Set")) -> ()  [unwired: 6 in, 3 out]
        n162 = call "Hide Animated Busy Icon with Message and Abort Button.vi"("Message"="Conversion aborted.", "Error In"=errorcluster {"status"=FALSE, "code"=0, "source"=""}) -> ("Error Out"=w591:errorcluster)  [unwired: 17 in]
        n163 = call "Current Date & Time String (High Precision).vi"() -> ("time string"=w587:string, "date string"=w588:string)  [unwired: 8 in, 2 out]
        n164 = Format Into String(format string="Conversion aborted on %s at %s" ("Message"), error in=w591, w588, w587) -> (resulting string=w577:string, error out=w592:errorcluster)  [unwired: 1 in]
      }
    }
    n165 = call "Send Message to Notebook.vi"("Error In"=w49, "Message"=w50, "Notebook Queue"=w52) -> ("Error Out"=w48:errorcluster, "Notebook Queue"=w51:refnum<queue>)  [unwired: 5 in]
    n166 = call "Message Style.vi"() -> ()  [unwired: 1 out]
    n167 = call "Send Error to Notebook.vi"("error in (no error)"=w48, "Notebook Q"=w51) -> ()  [unwired: 9 in, 1 out]
  }
  n168 = call <vilib>:"Destructor.vi"("BalloonTip in"=w33) -> ("error out"=w7:errorcluster)  [unwired: 10 in]
  n169 = Unregister For Events(event registration refnum=w32, error in=w31) -> (error out=w18:errorcluster)
  n170 = Merge Errors(w7, w18) -> (w8:errorcluster)
  n171 = call "Clear Error.vi"("Error In"=w8) -> ("no Error Out"=w17:errorcluster)  [unwired: 8 in]
  n172 = call "Alligator Variables Storage.vi"("Get(F)/Set"=w11, "AlliGator Variable"=AlliGator_Variables_List."Frames in Dataset" ("Alligator Variable"), "Error In"=w17, "Data in"=w14) -> ("Error Out"=w16:errorcluster)  [unwired: 5 in, 2 out]
  n173 = call "Alligator Variables Storage.vi"("Get(F)/Set"=w11, "AlliGator Variable"=AlliGator_Variables_List."Current Frame in Dataset" ("Alligator Variable"), "Error In"=w16, "Data in"=w14) -> ("Error Out"=w13:errorcluster)  [unwired: 5 in, 2 out]
  n174 = call "Alligator Variables Storage.vi"("Get(F)/Set"=w11, "AlliGator Variable"=AlliGator_Variables_List."Current Frame Timestamp" ("Alligator Variable"), "Error In"=w13, "Data in"=nan) -> ("Error Out"=w9:errorcluster)  [unwired: 5 in, 2 out]
  n175 = property on="Conversion Jobs" class="Arr"(error in=w9, "Value"=w46) -> (error out=w42:errorcluster)  [unwired: 1 in, 1 out]
  n176 = invoke class="VI" method="FP.Close"(error in=w42) -> (reference out=w21:refnum<vi>, error out=w20:errorcluster)  [unwired: 2 in, 1 out]
  n177 = Close Reference(reference=w21, error in (no error)=w20) -> ()  [unwired: 1 out]
  "Message" <- ""
